vi "Check P2.vi"(5 "Calibrated Results (P2 Hole)":sgl, 7 "Calibrated Results (P2 Right Edge Angle)":sgl, 9 "Calibrated Results (P2 Left Edge Angles)":sgl) -> (2 "P2 Status":bool, 6 "P2 Hole Status":bool, 8 "P2 Left Edge Angle Status":bool, 10 "P2 Right Edge Angle Status":bool)   [LabVIEW 2020]
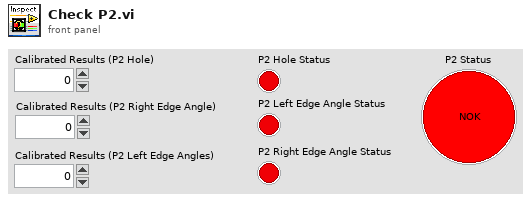
[diagram p1: front panel]
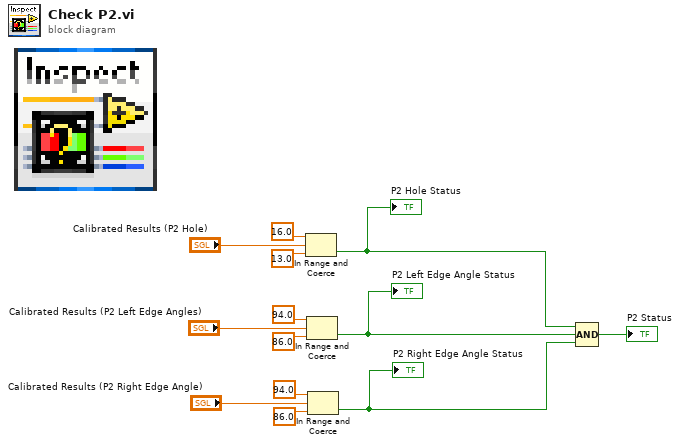
[diagram p0: block diagram]
diagram:
  n1 = In Range and Coerce(upper limit=16.0, x="Calibrated Results (P2 Hole)", lower limit=13.0) -> (In Range?=w6:bool)  [unwired: 1 out]
  "P2 Hole Status" <- w6
  n2 = In Range and Coerce(upper limit=94.0, x="Calibrated Results (P2 Left Edge Angles)", lower limit=86.0) -> (In Range?=w5:bool)  [unwired: 1 out]
  "P2 Left Edge Angle Status" <- w5
  n3 = In Range and Coerce(upper limit=94.0, x="Calibrated Results (P2 Right Edge Angle)", lower limit=86.0) -> (In Range?=w4:bool)  [unwired: 1 out]
  "P2 Right Edge Angle Status" <- w4
  n4 = Compound Arithmetic op=AND(w6, w5, w4) -> (→"P2 Status":bool)
